vi "ex_4_3_v2.vi"() -> ()   [LabVIEW 2020]
uses:
  <vilib>/numeric/Random Number (Range) DBL.vi
panel:
  out "Mean":dbl
  out "Array B":dbl[][](array[numeric])
  in  "Input number":dbl
  in  "Column number":i32
  in  "Row number":i32
  out "Array A":dbl[][](array[numeric])
  out "Array":dbl[][](array[numeric])
  in  "N":i32
  in  "M":i32
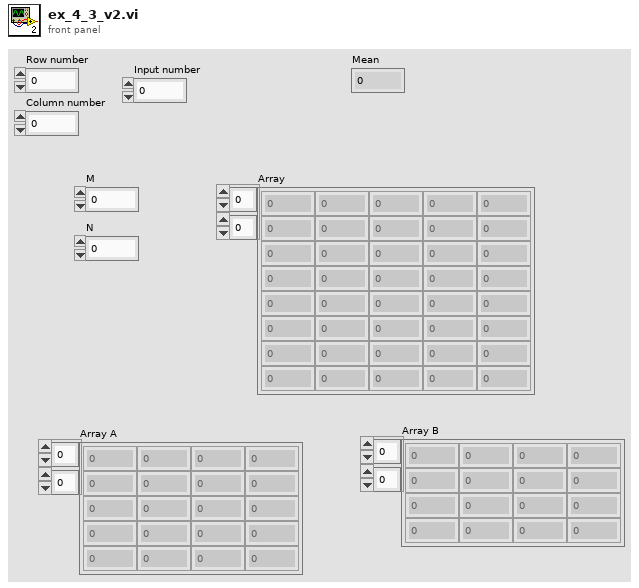
[diagram p1: front panel]
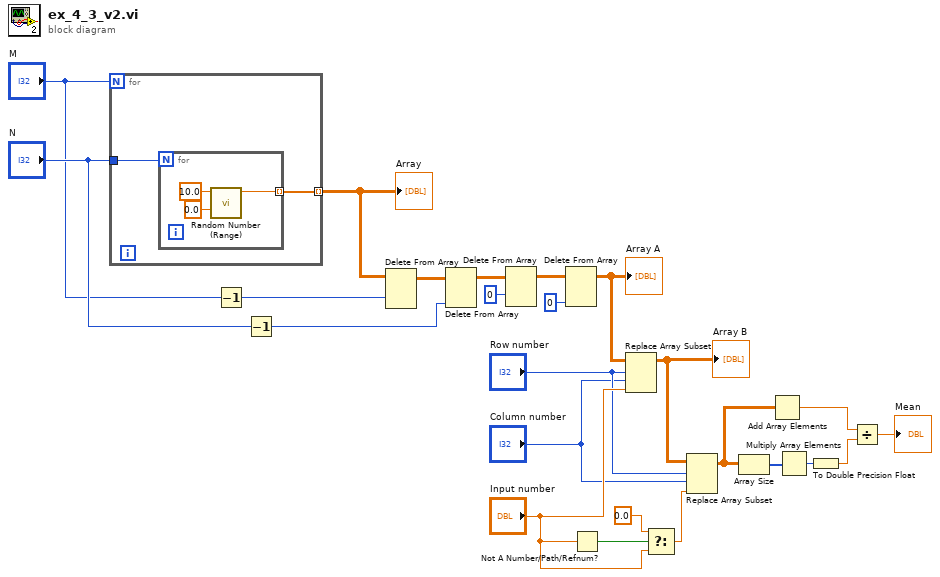
[diagram p0: block diagram]
diagram:
  n1 = for {
    N: "M" -> [_]
    tunnel: "N" -> [w26]
    tunnel: [w25] -> w22 mode=indexing
    n2 = for {
      N: w26 -> [_]
      tunnel: [w29] -> w25 mode=indexing
      n3 = call-poly <vilib>:"Random Number (Range).vi"("lower bound (0)"=0.0, "upper bound (100)"=10.0) -> ("number"=w29:dbl)  [unwired: 9 in]
    }
  }
  "Array" <- w22
  n4 = Decrement(x="M") -> (x-1=w18:i32)
  n5 = Decrement(x="N") -> (x-1=w17:i32)
  n6 = Delete From Array(array=w22, index (row)=w18) -> (array with subset deleted=w21:dbl[][])  [unwired: 2 in, 1 out]
  n7 = Delete From Array(array=w21, index (col)=w17) -> (array with subset deleted=w20:dbl[][])  [unwired: 2 in, 1 out]
  n8 = Delete From Array(array=w20, index (row)=0) -> (array with subset deleted=w19:dbl[][])  [unwired: 2 in, 1 out]
  n9 = Delete From Array(array=w19, index (col)=0 ("disabled index (col)")) -> (array with subset deleted=w14:dbl[][])  [unwired: 2 in, 1 out]
  "Array A" <- w14
  n10 = Not A Number/Path/Refnum?(number/path/refnum="Input number") -> (NaN/Path/Refnum?=w7:bool)
  n11 = Replace Array Subset(array=w14, new element="Input number", index (row)="Row number", index (col)="Column number") -> (w8:dbl[][])
  "Array B" <- w8
  n12 = Select(t=0.0 ("f"), s=w7, f="Input number") -> (s? t:f=w2:dbl)
  n13 = Replace Array Subset(array=w8, new element=w2, index (row)="Row number", index (col)="Column number") -> (w1:dbl[][])
  n14 = Array Size(array=w1) -> (size(s)=w13:i32[])
  n15 = Add Array Elements(numeric array=w1) -> (sum=w11:dbl)
  n16 = Multiply Array Elements(1:w13) -> (0:w12:i32)
  n17 = To Double Precision Float(number=w12) -> (double precision float=w10:dbl)
  n18 = Divide(x=w11, y=w10) -> (x/y=→"Mean":dbl)
